vi "Add .NET Event Callback Refnum.vi"(9 "Event Callback Refnum":refnum<k27>, 10 "Event Name":string="Click", 11 "MyEventGrid in":refnum<class "MyEventGrid.lvclass">) -> (3 "MyEventGrid out":refnum<class "MyEventGrid.lvclass">)   [LabVIEW 2024, in "MyEventGrid.lvclass"]
uses:
  MyEventGrid.lvclass
  MyEventGrid.lvclass/MyEventGrid.ctl
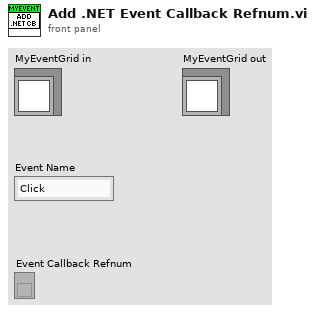
[diagram p1: front panel]
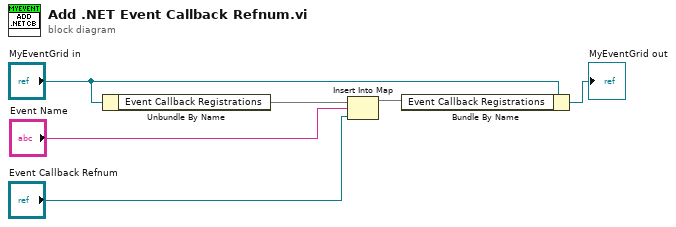
[diagram p0: block diagram]
diagram:
  n1 = Unbundle By Name("MyEventGrid in") -> ("Event Callback Registrations"=w6:map{string, refnum<k27>})
  n2 = Insert Into Map(map in=w6, key="Event Name", value="Event Callback Refnum") -> (map out=w4:map{string, refnum<k27>})  [unwired: 2 out]
  n3 = Bundle By Name(cluster="MyEventGrid in", "Event Callback Registrations"=w4) -> (→"MyEventGrid out":refnum<class "MyEventGrid.lvclass">)
